vi "SECoP_dataCreateBool.vi"(6 "bValue":bool, 8 "error in (no error)":errorcluster, 11 "DLL path (in)":T2) -> (0 "error out":errorcluster, 2 "SECoP_dataPtr (out)":T1 {"ptr64" format="%.0x"; "ptr32" format="%.0x"}, 3 "DLL path (out)":T2)   [LabVIEW 2023, in "SECoP.lvlib"]
doc: "Call <b>\"SECoP_dataCreateBool.vi\"</b> to create a simple boolean data type and set value. Free resources after use with <b>\"SECoP_dataDestroy.vi\"</b>.\n\n<b>DLL path</b> input and output of cluster from \"SECoP-Initialize.vi\"\n<b>bValue</b> new value\n<b>SECoP_dataPtr</b> created data"
uses:
  SECoP.lvlib
  SECoP-libraries.ctl
  SECoP-data.ctl
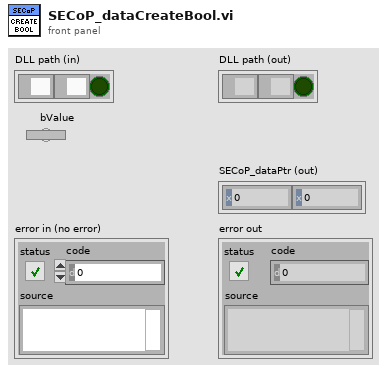
[diagram p1: front panel]
types:
  T1 = typedef "SECoP.lvlib/SECoP-data.ctl" = cluster{"ptr32":u32, "ptr64":u64}
  T2 = typedef "SECoP.lvlib/SECoP-libraries.ctl" = cluster{"serverDLL":path, "variantDLL":path, "cleanup_mode":bool}
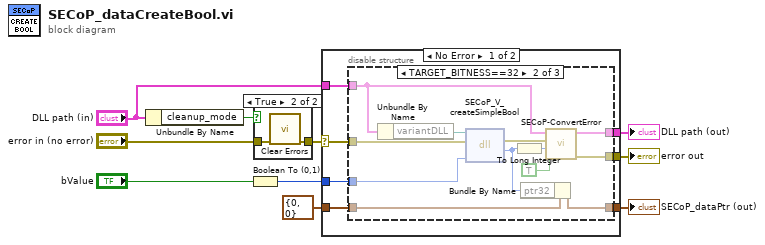
[diagram p0: block diagram]
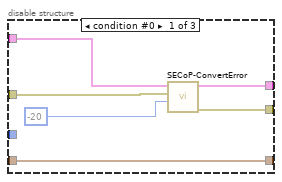
[diagram p3: hidden frame]
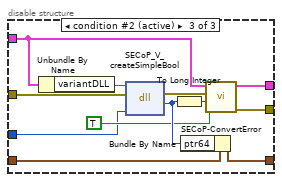
[diagram p4: hidden frame]
diagram:
  n1 = Unbundle By Name("DLL path (in)") -> ("cleanup_mode"=w8:bool)
  n2 = Boolean To (0,1)(Boolean="bValue") -> (0, 1=w1:i16)
  n3 = case shown="True" w8 {
    tunnel: "error in (no error)" -> [w11 w13]
    tunnel: [w11 w12] -> w6
    frame False {
    }
    frame True {
      n4 = call <vilib>:"Clear Errors.vi"("error in (no error)"=w13) -> ("error out"=w12:errorcluster)  [unwired: 5 in, 1 out]
    }
  }
  n5 = case shown="No Error" w6 {
    selector: w6 -> [w20 w52]
    tunnel: "DLL path (in)" -> [w19 w53]
    tunnel: [w17 w53] -> w10
    tunnel: [w18 w52] -> w9
    tunnel: [w15 w51] -> w5
    tunnel: T1 {"ptr32"=0, "ptr64"=0} ("SECoP_dataPtr (out)") -> [w16 w51]
    tunnel: w1 -> [w14 _]
    frame No Error {
      n6 = disable-structure shown="TARGET_BITNESS==32" {
        disable-tunnel: w20 -> [w26 w38 w50]
        disable-tunnel: w19 -> [w25 w27 w39]
        disable-tunnel: [w23 w34 w46] -> w18
        disable-tunnel: [w24 w33 w45] -> w17
        disable-tunnel: w16 -> [w21 w36 w48]
        disable-tunnel: [w21 w37 w49] -> w15
        disable-tunnel: w14 -> [_ w29 w41]
        frame condition #0 {
          n7 = call "SECoP-ConvertError.vi"("return code"=-20, "error in (no error)"=w26, "DLL path (in)"=w25) -> ("error out"=w23:errorcluster, "DLL path (out)"=w24:T2)  [unwired: 7 in]
        }
        frame condition #1 {
          n8 = Unbundle By Name(w27) -> ("variantDLL"=w28:path)
          n9 = dll-call lib="Z:/Praktische_Aufgaben/SECoP-LabVIEW2015/32bit/SECoP32.dll" fn="SECoP_V_createSimpleBool"(path in=w28, error in=w38, "bValue"=w29) -> (error out=w35:errorcluster, "return type"=w32:u32)  [unwired: 2 in, 1 out]
          n10 = To Long Integer(number=w32) -> (32bit integer=w30:i32)
          n11 = Bundle By Name(cluster=w36, "ptr32"=w32) -> (w37:T1)
          n12 = call "SECoP-ConvertError.vi"("return is boolean"=TRUE, "return code"=w30, "error in (no error)"=w35, "DLL path (in)"=w27) -> ("error out"=w34:errorcluster, "DLL path (out)"=w33:T2)  [unwired: 6 in]
        }
        frame condition #2 (active) {
          n13 = Unbundle By Name(w39) -> ("variantDLL"=w40:path)
          n14 = dll-call lib="Z:/Praktische_Aufgaben/SECoP-LabVIEW2015/32bit/SECoP32.dll" fn="SECoP_V_createSimpleBool"(path in=w40, error in=w50, "bValue"=w41) -> (error out=w47:errorcluster, "return type"=w44:u64)  [unwired: 2 in, 1 out]
          n15 = To Long Integer(number=w44) -> (32bit integer=w42:i32)
          n16 = Bundle By Name(cluster=w48, "ptr64"=w44) -> (w49:T1)
          n17 = call "SECoP-ConvertError.vi"("return is boolean"=TRUE, "return code"=w42, "error in (no error)"=w47, "DLL path (in)"=w39) -> ("error out"=w46:errorcluster, "DLL path (out)"=w45:T2)  [unwired: 6 in]
        }
      }
    }
    frame Error {
    }
  }
  "DLL path (out)" <- w10
  "error out" <- w9
  "SECoP_dataPtr (out)" <- w5
